vi "QueryFirst.vi"(6 "commandTimeout in":i32=-1, 7 "CommandType":i32(ring)=-1 items=["Text"=1, "StoredProcedure"=4, "TableDirect"=512], 8 "error in (no error)":errorcluster, 9 "DynamicParameters in":refnum<class "DynamicParameters.lvclass">, 10 "sql":string, 11 "SqlMapper in":refnum<class "SqlMapper.lvclass">) -> (0 "error out":errorcluster, 2 "Value":variant, 3 "SqlMapper out":refnum<class "SqlMapper.lvclass">)   [LabVIEW 2020, in "ORM.lvlib" / "SqlMapper.lvclass"]
uses:
  SqlMapper.lvclass
  DynamicParameters/DynamicParameters.lvclass
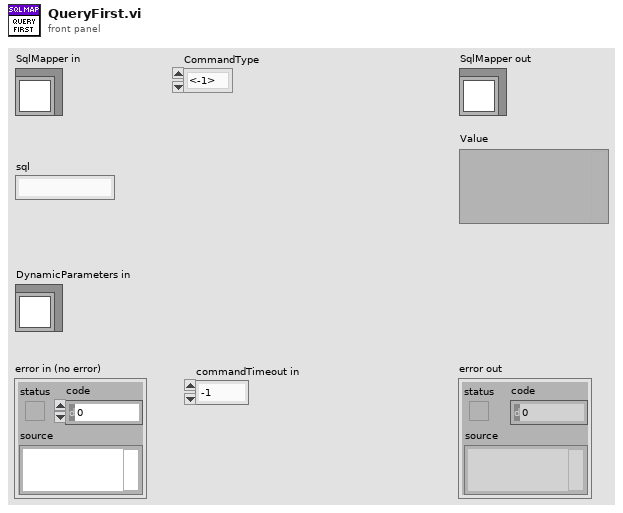
[diagram p1: front panel]
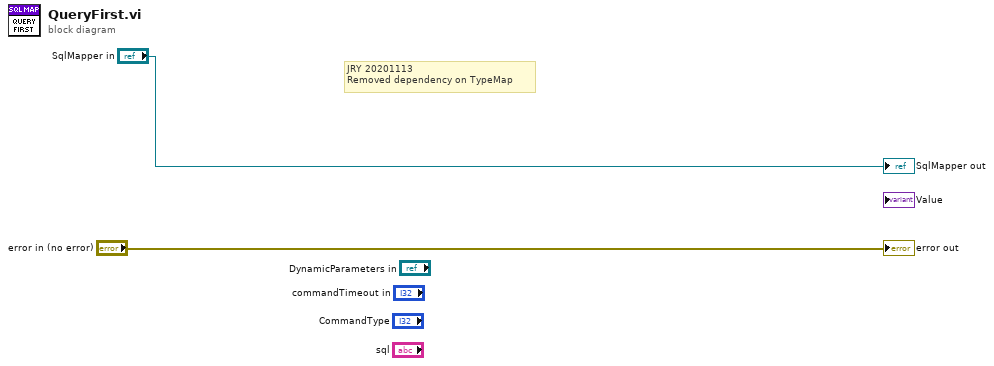
[diagram p0: block diagram]
diagram:
  # "JRY 20201113\nRemoved dependency on TypeMap"
  "error out" <- "error in (no error)"
  "SqlMapper out" <- "SqlMapper in"
